vi "发送数据打包-八位校验和.vi"(8 "16进制字符串":string, 10 "命令数":u8) -> (0 "结果字符串":string, 1 "校验和":u8)   [LabVIEW 2016]
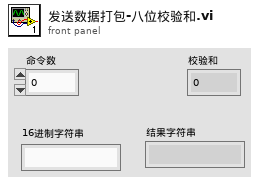
[diagram p1: front panel]
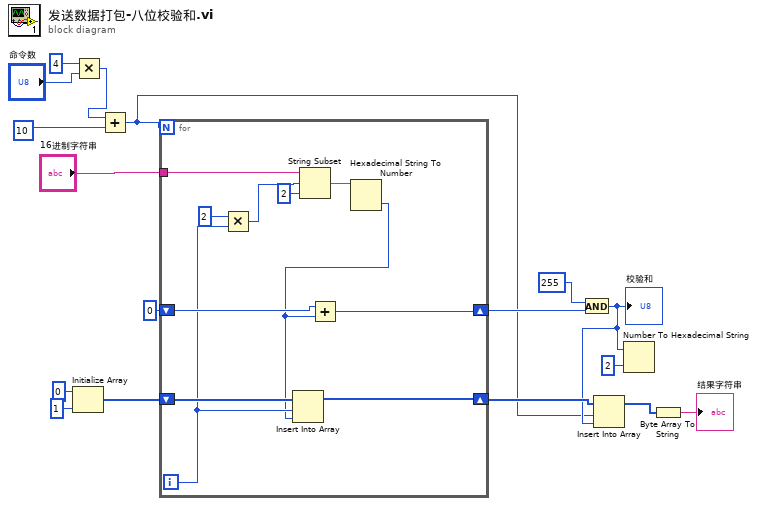
[diagram p0: block diagram]
diagram:
  n1 = Initialize Array(u8 0 ("元素"), 1 ("维数大小")) -> (w11:u8[])
  n2 = Multiply(x=u8 4, y="命令数") -> (x*y=w1:u8)
  n3 = Add(x=w1, y=u8 10) -> (x+y=w6:u8)
  n4 = for {
    N: w6 -> [_]
    tunnel: "16进制字符串" -> [w28]
    shift-right: [w22] -> w13
    shift-left: u32 0 -> [w23]
    shift-right: [w18] -> w8
    shift-left: w11 -> [w21]
    i -> [w20]
    n5 = Multiply(x=2, y=w20) -> (x*y=w26:i32)
    n6 = String Subset(string=w28, offset (0)=w26, length (rest)=2 ("长度（剩余）")) -> (substring=w24:string)
    n7 = Hexadecimal String To Number(string=w24) -> (number=w19:u32)  [unwired: 2 in, 1 out]
    n8 = Insert Into Array(array=w21, index=w20, new element=w19) -> (w18:u8[])
    n9 = Add(x=w23, y=w19) -> (x+y=w22:u32)
  }
  n10 = And(x=u8 255, y=w13) -> (x .and. y?=w7:u32)
  "校验和" <- w7
  n11 = Insert Into Array(array=w8, index=w6, new element=w7) -> (w5:u8[])
  n12 = Number To Hexadecimal String(1:i16 2 ("宽度(-)"), 2:w7) -> ()  [unwired: 1 out]
  n13 = Byte Array To String(unsigned byte array=w5) -> (string=→"结果字符串":string)
